vi "Created Events.vi"(8 "Created Event Alias":string, 9 "Priority?":bool, 10 "Msg Strategy":refnum<class "Msg Strategy.lvclass">, 11 "Template Queue in":refnum<class "Template Queue.lvclass">) -> (3 "Template Queue out":refnum<class "Template Queue.lvclass">)   [LabVIEW 2021, in "_Template.lvlib" / "Templates.lvlib" / "Template Queue.lvlib" / "Template Queue.lvclass"]
uses:
  Template Queue.lvclass
  <vilib>/jettl/jettl/jettl/Msg Strategy/Msg Strategy.lvclass
  Template Queue.lvclass/Template Queue.ctl
  <vilib>/jettl/jettl/jettl/Queue/Queue.lvclass
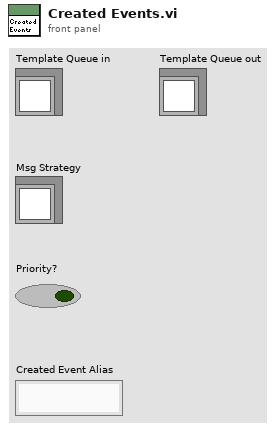
[diagram p1: front panel]
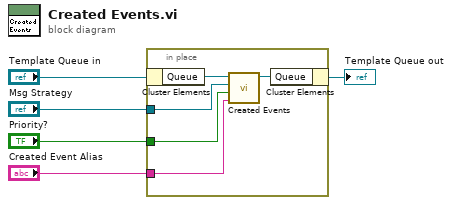
[diagram p0: block diagram]
diagram:
  n1 = in-place {
    in-place-border: "Msg Strategy" -> [w8]
    in-place-border: "Priority?" -> [w7]
    in-place-border: "Created Event Alias" -> [w6]
    n2 = in-place-cluster #1("Template Queue in") -> ("Queue"=w10:refnum<class "Queue.lvclass">)
    n3 = call-dynamic "Created Events.vi"("Created Event Alias"=w6, "Priority?"=w7, "Msg Strategy"=w8, "Queue in"=w10) -> ("Queue out"=w9:refnum<class "Queue.lvclass">)  [unwired: 7 in]
    n4 = in-place-cluster #1("Queue"=w9) -> (→"Template Queue out":refnum<class "Template Queue.lvclass">)
  }
